vi "cursor window action stack.vi"(7 "stack action":T2, 8 "action list":T1[](array[typedef]), 9 "cursor window action":T1=enum."check", 11 "command stack":T1[](array[typedef])) -> (1 "cursor window action out":T1=enum."check", 2 "stack is empty ?":bool, 3 "command stack out":T1[](array[typedef]))   [LabVIEW 2021]
uses:
  stack action -- control.ctl
  cursor window action.ctl
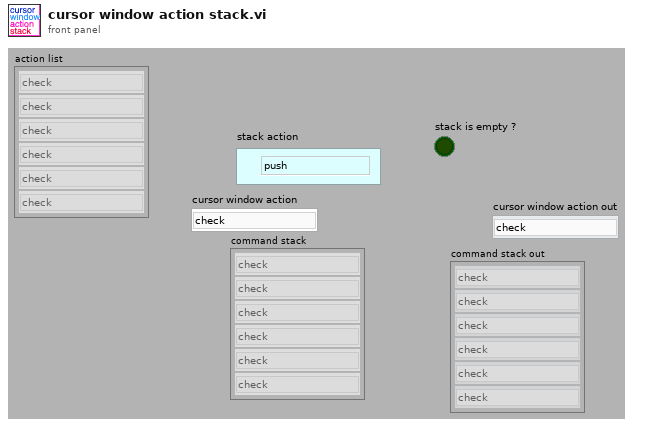
[diagram p1: front panel]
types:
  T1 = typedef "cursor window action.ctl" = enum16{"balance", "h. offset change", "cursor moves", "change center", "change window", "init", "check", "reset", "set y to middle", "idle", "-write all Y", "-write left.X", "-write center.X", "-write right.X", "-write all X", "-change center", "-change window", "-change skew", "-read cursor 2", "-read cursor 1", "-read cursor 0", "-read all cursors", "-reset", "-read plot scale", "-set y to middle", "-Q: center.Y is visible", "-Q: window is visible", "-parse center.Y", "-right left from center", "-left move", "-right move", "-set center.Y", "-empty", "-set cursors to default", "-check", "-write center.Y", "-copy cursor 1", "-copy cursor 0", "-copy cursor 2", "move right", "move left", "shrink", "broaden", "skew up", "skew down", "-write plot scale", "zoom X", "change cen&win", "zoom to all data", "color--red", "color--green", "color--yellow", "read", "zoom out", "zoom in", "slide right", "slide left", "set range aspect ratio to 1", "move to window range", "--move to window range"}
  T2 = typedef "stack action -- control.ctl" = enum16{"push", "pop", "check", "init"}
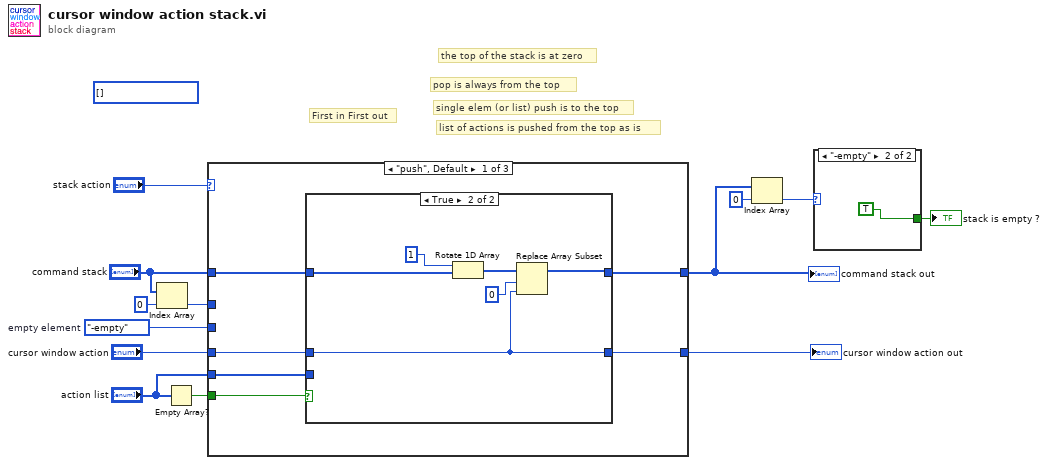
[diagram p0: block diagram]
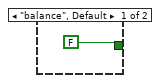
[diagram p2: hidden frame]
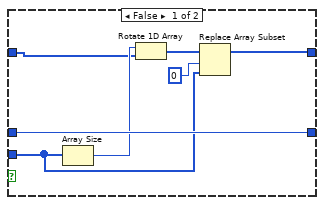
[diagram p3: hidden frame]
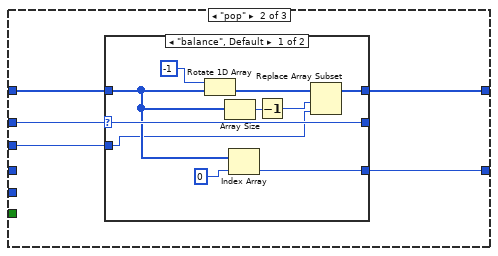
[diagram p4: hidden frame]
diagram:
  w1 = cursor_window_action."-empty"  # empty element
  (unwired) T1[] [] items=["balance", "h. offset change", "cursor moves", "change center", "change window", "init", "check", "reset", "set y to middle", "idle", "-write all Y", "-write left.X", "-write center.X", "-write right.X", "-write all X", "-change center", "-change window", "-change skew", "-read cursor 2", "-read cursor 1", "-read cursor 0", "-read all cursors", "-reset", "-read plot scale", "-set y to middle", "-Q: center.Y is visible", "-Q: window is visible", "-parse center.Y", "-right left from center", "-left move", "-right move", "-set center.Y", "-empty", "-set cursors to default", "-check", "-write center.Y", "-copy cursor 1", "-copy cursor 0", "-copy cursor 2", "move right", "move left", "shrink", "broaden", "skew up", "skew down", "-write plot scale", "zoom X", "change cen&win", "zoom to all data", "color--red", "color--green", "color--yellow", "read", "zoom out", "zoom in", "slide right", "slide left", "set range aspect ratio to 1", "move to window range", "--move to window range"] ("command stack")
  # "list of actions is pushed from the top as is"
  # "single elem (or list) push is to the top"
  # "pop is always from the top"
  # "First in First out"
  # "the top of the stack is at zero"
  n1 = Index Array(array="command stack", index=0) -> (element=w6:T1)
  n2 = Empty Array?(array="action list") -> (empty?=w10:bool)
  n3 = case shown="\"push\", Default" "stack action" {
    tunnel: [w19 w37 w51] -> w4
    tunnel: "command stack" -> [w18 w36 w51]
    tunnel: w6 -> [_ w35 _]
    tunnel: [w14 w34 w52] -> w11
    tunnel: "cursor window action" -> [w17 _ w52]
    tunnel: w10 -> [w16 _ _]
    tunnel: "action list" -> [w15 _ _]
    tunnel: w1 -> [_ w33 _]
    frame "push", Default {
      n4 = case shown="True" w16 {
        tunnel: [w20 w27] -> w19
        tunnel: w18 -> [w24 w29]
        tunnel: w17 -> [w26 w30]
        tunnel: w15 -> [w21 _]
        tunnel: [w26 w30] -> w14
        frame False {
          n5 = Array Size(array=w21) -> (size(s)=w25:i32)
          n6 = Rotate 1D Array(1:w24, 2:w25) -> (0:w23:T1[])
          n7 = Replace Array Subset(array=w23, new element=w21, index=0) -> (w20:T1[])
        }
        frame True {
          n8 = Rotate 1D Array(1:w29, 2:1) -> (0:w32:T1[])
          n9 = Replace Array Subset(array=w32, new element=w30, index=0) -> (w27:T1[])
        }
      }
    }
    frame "pop" {
      n10 = case shown="\"balance\", Default" w35 {
        selector: w35 -> [w45 w49]
        tunnel: [w41 w50] -> w37
        tunnel: w36 -> [w42 w50]
        tunnel: [w46 w48] -> w34
        tunnel: [w45 w49] -> _
        tunnel: w33 -> [w38 w48]
        frame "balance", Default {
          n11 = Rotate 1D Array(1:w42, 2:-1) -> (0:w40:T1[])
          n12 = Array Size(array=w42) -> (size(s)=w43:i32)
          n13 = Index Array(array=w42, index=0) -> (element=w46:T1)
          n14 = Decrement(x=w43) -> (x-1=w39:i32)
          n15 = Replace Array Subset(array=w40, new element=w38, index=w39) -> (w41:T1[])
        }
        frame "-empty" {
        }
      }
    }
    frame "check" {
    }
  }
  "command stack out" <- w4
  "cursor window action out" <- w11
  n16 = Index Array(array=w4, index=0) -> (element=w3:T1)
  n17 = case shown="\"-empty\"" w3 {
    tunnel: [FALSE TRUE] -> w2
    frame "balance", Default {
    }
    frame "-empty" {
    }
  }
  "stack is empty ?" <- w2
